vi "Initialize.vi"(8 "error in (no error)":errorcluster, 10 "motorSettings":T1={"maxVelocity"=0.0, "acceleration"=0.0, "maxTravel"=0.0, "minTravel"=0.0, "waitTimeout"=0, "stageType"=32, "units"="", "homeConfig"={"direction"=1, "limitSwitch"=0, "offsetDistance"=0.0, "velocity"=0.0, "waitTimeout"=0, "postHomeTravel"=0.0}, "jogSettings"={"jogSize"=0.0, "maxVelocity"=0.0, "acceleration"=0.0, "waitTimeout"=0}, "Setup Offset"=0.0} {"stageType" items=["ZST6"=32, "ZST13"=33, "ZST25"=34, "ZST206"=48, "ZST213"=49, "ZST225"=50, "ZFS206"=64, "ZFS213"=65, "ZFS225"=66, "NR360"=112, "PLS_X25MM"=114, "PLS_X25MM_HiRes"=115, "FW103"=117]; "homeConfig"."limitSwitch" items=["Ignore"=0, "ClockwiseHard"=1, "CounterClockwiseHard"=4]; "homeConfig"."direction" items=["Clockwise"=1, "CounterClockwise"=2]}, 11 "serialNumber":string) -> (0 "error out":errorcluster, 3 "KST101 out":refnum<class "KST101.lvclass">)   [LabVIEW 2016, in "Stepper Motor Controller.lvlib" / "KST101.lvclass"]
uses:
  KST101.lvclass
  TypeDefs/KST-MotorSettings.ctl
  TypeDefs/KST-HomeConfig.ctl
  TypeDefs/KST-JogConfig.ctl
  KST101.lvclass/KST101.ctl
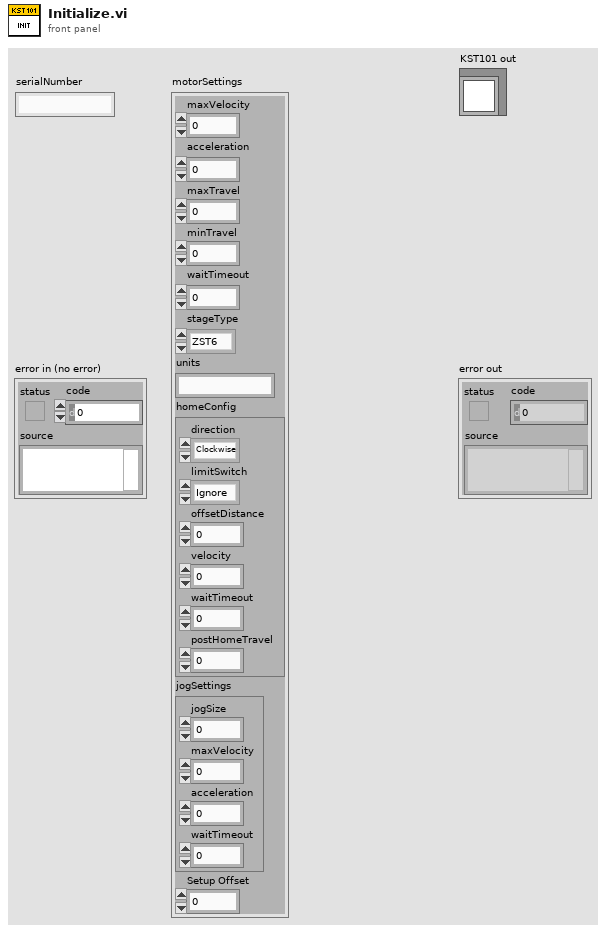
[diagram p1: front panel]
types:
  T1 = typedef "Stepper Motor Controller.lvlib/KST101.lvclass/KST-MotorSettings.ctl" = cluster{"maxVelocity":dbl, "acceleration":dbl, "maxTravel":dbl, "minTravel":dbl, "waitTimeout":i32, "stageType":i32, "units":string, "homeConfig":T2, "jogSettings":T3, "Setup Offset":dbl}
  T2 = typedef "Stepper Motor Controller.lvlib/KST101.lvclass/KST-HomeConfig.ctl" = cluster{"direction":i32, "limitSwitch":i32, "offsetDistance":dbl, "velocity":dbl, "waitTimeout":i32, "postHomeTravel":dbl}
  T3 = typedef "Stepper Motor Controller.lvlib/KST101.lvclass/KST-JogConfig.ctl" = cluster{"jogSize":dbl, "maxVelocity":dbl, "acceleration":dbl, "waitTimeout":i32}
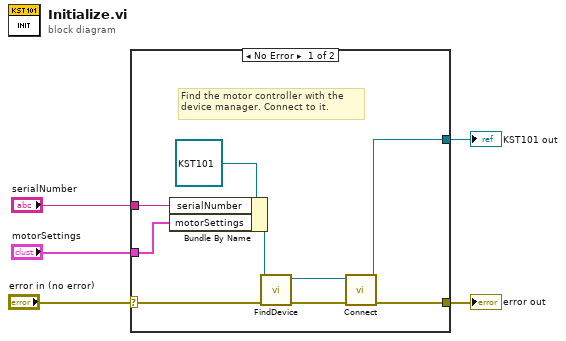
[diagram p0: block diagram]
diagram:
  n1 = case shown="No Error" "error in (no error)" {
    selector: "error in (no error)" -> [w10 w15]
    tunnel: [w9 w15] -> w4
    tunnel: [w7 _] -> w3
    tunnel: "serialNumber" -> [w14 _]
    tunnel: "motorSettings" -> [w13 _]
    frame No Error {
      # "Find the motor controller with the \ndevice manager. Connect to it."
      n2 = Bundle By Name(cluster=refnum<class "KST101.lvclass"> refnum ("KST101 in"), "serialNumber"=w14, "motorSettings"=w13) -> (w8:refnum<class "KST101.lvclass">)
      n3 = call-dynamic "FindDevice.vi"("error in (no error)"=w10, "KST101 in"=w8) -> ("error out"=w11:errorcluster, "KST101 out"=w12:refnum<class "KST101.lvclass">)  [unwired: 8 in]
      n4 = call-dynamic "Connect.vi"("error in (no error)"=w11, "KST101 in"=w12) -> ("error out"=w9:errorcluster, "KST101 out"=w7:refnum<class "KST101.lvclass">)  [unwired: 8 in]
    }
    frame Error {
    }
  }
  "error out" <- w4
  "KST101 out" <- w3
